vi "CH0_LCD_to_PC_display_correction.vi"(6 "n_Shift 1":dbl, 7 "CH0_range_in":u8, 8 "p_Shift 1":dbl, 9 "n_Gain 1":dbl=1.0, 10 "p_Gain 1":dbl=1.0, 11 "Vin":dbl) -> (3 "Vout":dbl)   [LabVIEW 2012]
panel:
  in  "p_Shift 10":dbl
  in  "n_Shift 10":dbl
  in  "n_Gain 10":dbl=1.0
  in  "p_Gain 10":dbl=1.0
  in  "p_Shift 80":dbl
  in  "n_Shift 80":dbl
  in  "n_Gain 80":dbl=1.0
  in  "p_Gain 80":dbl=1.0
  in  "p_Shift 51":dbl
  in  "n_Shift 51":dbl
  in  "n_Gain 51":dbl=1.0
  in  "p_Gain 51":dbl=1.0
  # "CH0"
  # "+/-9V"
  # "+/-55V"
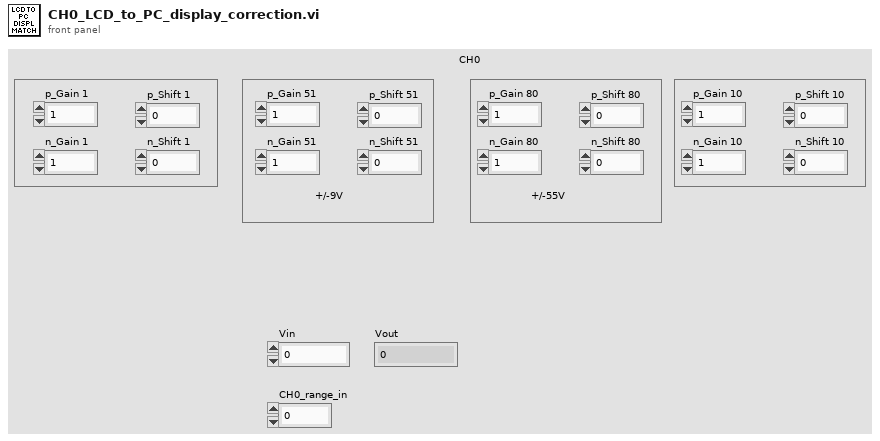
[diagram p1: front panel]
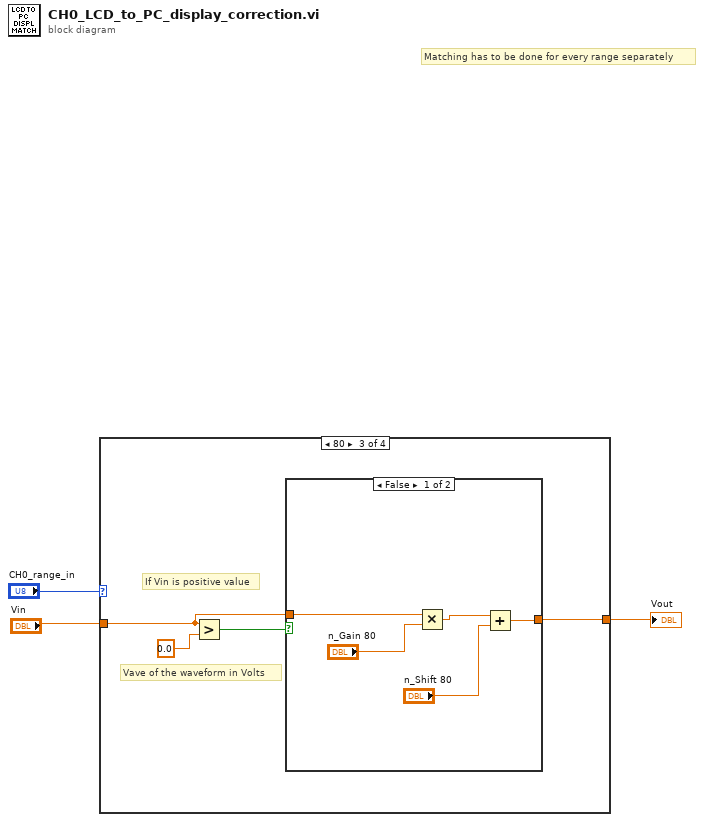
[diagram p0: block diagram]
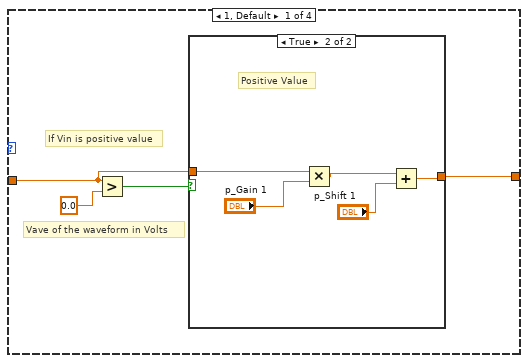
[diagram p2: hidden frame]
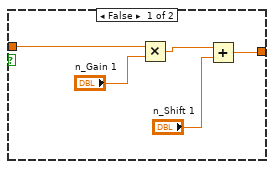
[diagram p3: hidden frame]
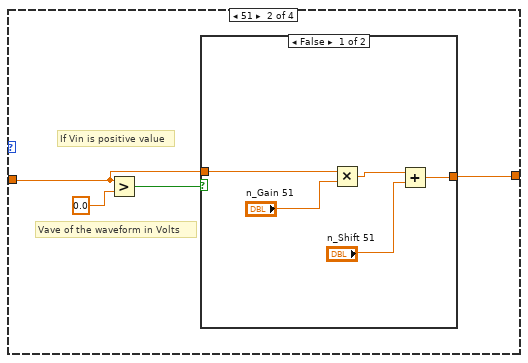
[diagram p4: hidden frame]
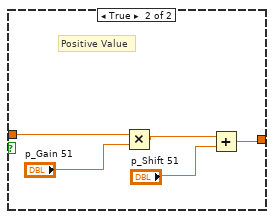
[diagram p5: hidden frame]
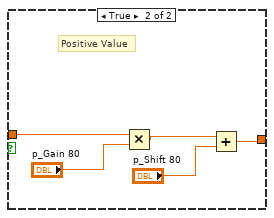
[diagram p6: hidden frame]
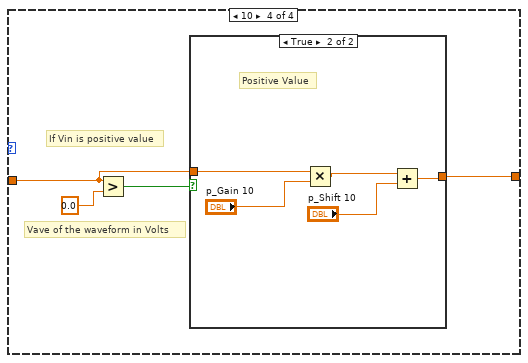
[diagram p7: hidden frame]
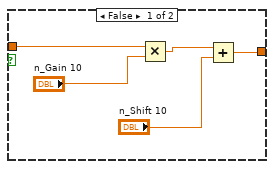
[diagram p8: hidden frame]
diagram:
  # "Matching has to be done for every range separately"
  n1 = case shown="80" "CH0_range_in" {
    tunnel: "Vin" -> [w5 w19 w33 w47]
    tunnel: [w4 w18 w32 w46] -> w1
    frame 1, Default {
      # "Vave of the waveform in Volts"
      # "If Vin is positive value"
      n2 = Greater?(x=w5, y=0.0) -> (0:w7:bool)
      n3 = case shown="True" w7 {
        tunnel: [w10 w14] -> w4
        tunnel: w5 -> [w11 w17]
        frame False {
          n4 = Multiply(x=w11, y="n_Gain 1") -> (x*y=w9:dbl)
          n5 = Add(x=w9, y="n_Shift 1") -> (x+y=w10:dbl)
        }
        frame True {
          # "Positive Value"
          n6 = Multiply(x=w17, y="p_Gain 1") -> (x*y=w13:dbl)
          n7 = Add(x=w13, y="p_Shift 1") -> (x+y=w14:dbl)
        }
      }
    }
    frame 51 {
      # "Vave of the waveform in Volts"
      # "If Vin is positive value"
      n8 = Greater?(x=w19, y=0.0) -> (0:w21:bool)
      n9 = case shown="False" w21 {
        tunnel: [w25 w30] -> w18
        tunnel: w19 -> [w26 w31]
        frame False {
          n10 = Multiply(x=w26, y="n_Gain 51") -> (x*y=w24:dbl)
          n11 = Add(x=w24, y="n_Shift 51") -> (x+y=w25:dbl)
        }
        frame True {
          # "Positive Value"
          n12 = Multiply(x=w31, y="p_Gain 51") -> (x*y=w29:dbl)
          n13 = Add(x=w29, y="p_Shift 51") -> (x+y=w30:dbl)
        }
      }
    }
    frame 80 {
      # "Vave of the waveform in Volts"
      # "If Vin is positive value"
      n14 = Greater?(x=w33, y=0.0) -> (0:w35:bool)
      n15 = case shown="False" w35 {
        tunnel: [w39 w44] -> w32
        tunnel: w33 -> [w40 w45]
        frame False {
          n16 = Multiply(x=w40, y="n_Gain 80") -> (x*y=w38:dbl)
          n17 = Add(x=w38, y="n_Shift 80") -> (x+y=w39:dbl)
        }
        frame True {
          # "Positive Value"
          n18 = Multiply(x=w45, y="p_Gain 80") -> (x*y=w43:dbl)
          n19 = Add(x=w43, y="p_Shift 80") -> (x+y=w44:dbl)
        }
      }
    }
    frame 10 {
      # "Vave of the waveform in Volts"
      # "If Vin is positive value"
      n20 = Greater?(x=w47, y=0.0) -> (0:w49:bool)
      n21 = case shown="True" w49 {
        tunnel: [w53 w58] -> w46
        tunnel: w47 -> [w54 w59]
        frame False {
          n22 = Multiply(x=w54, y="n_Gain 10") -> (x*y=w52:dbl)
          n23 = Add(x=w52, y="n_Shift 10") -> (x+y=w53:dbl)
        }
        frame True {
          # "Positive Value"
          n24 = Multiply(x=w59, y="p_Gain 10") -> (x*y=w57:dbl)
          n25 = Add(x=w57, y="p_Shift 10") -> (x+y=w58:dbl)
        }
      }
    }
  }
  "Vout" <- w1
